vi "Create.vi"(8 "ErrorIn":errorcluster, 11 "ReferenceIn":refnum<class "VerticalButtonBar.lvclass">) -> (0 "ErrorOut":errorcluster, 3 "ReferenceOut":refnum<class "VerticalButtonBar.lvclass">)   [LabVIEW 2021, in "VerticalButtonBar.lvclass"]
doc: "Create the object instance"
uses:
  VerticalButtonBar.lvclass
  VerticalButtonBar.lvclass/VerticalButtonBar.ctl
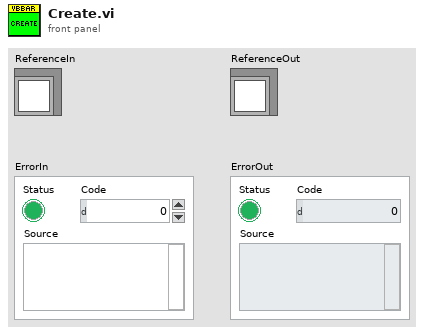
[diagram p1: front panel]
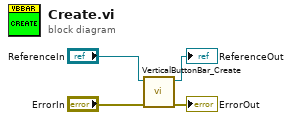
[diagram p0: block diagram]
diagram:
  n1 = call "VerticalButtonBar_Create.vi"("ErrorIn"="ErrorIn", "ReferenceIn"="ReferenceIn") -> ("ErrorOut"=→"ErrorOut":errorcluster, "ReferenceOut"=→"ReferenceOut":refnum<class "VerticalButtonBar.lvclass">)  [unwired: 8 in]
